vi "Build.vi"(8 "error in (no error)":errorcluster, 11 "CD Build Tools in":refnum<class "Project Sync Tools.lvclass">) -> (0 "error out":errorcluster, 3 "CD Build Tools out":refnum<class "Project Sync Tools.lvclass">)   [LabVIEW 2019]
uses:
  Project Sync Tools.lvclass
  <vilib>/AppBuilder/AB_API_Simple/NI_App_Builder_API.lvlib
  <vilib>/AppBuilder/AB_API_Simple/Build (path).vi
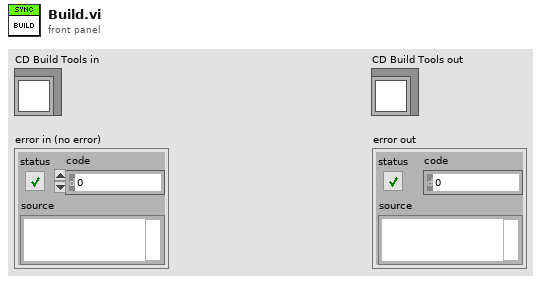
[diagram p1: front panel]
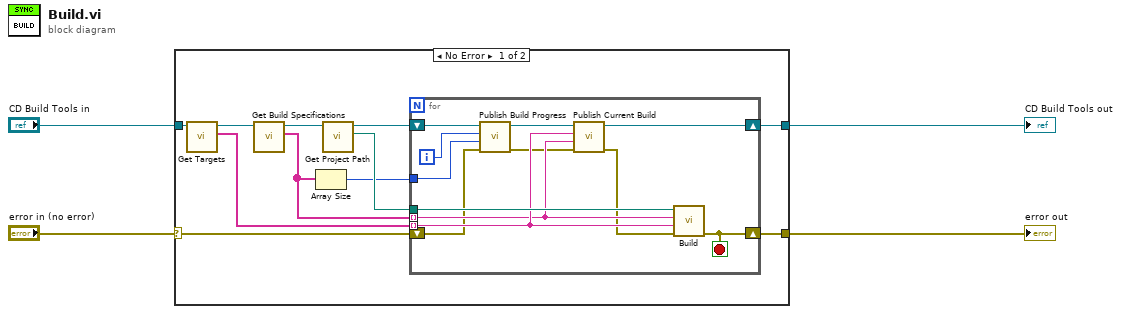
[diagram p0: block diagram]
diagram:
  n1 = case shown="No Error" "error in (no error)" {
    selector: "error in (no error)" -> [w9 w28]
    tunnel: [w5 w29] -> w1
    tunnel: [w13 w28] -> w2
    tunnel: "CD Build Tools in" -> [w12 w29]
    frame No Error {
      n2 = call "Get Targets.vi"("CD Build Tools in"=w12) -> ("Targets"=w10:string[], "CD Build Tools out"=w11:refnum<class "Project Sync Tools.lvclass">)  [unwired: 9 in]
      n3 = call "Get Build Specifications.vi"("CD Build Tools in"=w11) -> ("Build Specifications"=w8:string[], "CD Build Tools out"=w14:refnum<class "Project Sync Tools.lvclass">)  [unwired: 9 in]
      n4 = Array Size(array=w8) -> (size(s)=w7:i32)
      n5 = call "Get Project Path.vi"("CD Build Tools in"=w14) -> ("Project Path"=w15:path, "CD Build Tools out"=w6:refnum<class "Project Sync Tools.lvclass">)  [unwired: 9 in]
      n6 = for {
        tunnel: w15 -> [w27]
        shift-right: [w26] -> w13
        shift-left: w9 -> [w20]
        tunnel: w8 -> [w24] mode=indexing
        tunnel: w10 -> [w25] mode=indexing
        tunnel: w7 -> [w21]
        shift-right: [w17] -> w5
        shift-left: w6 -> [w23]
        i -> [w22]
        stop <- w26 stop-if-true
        n7 = call "Publish Build Progress.vi"("error in (no error)"=w20, "Total Number of Builds"=w21, "Current Iteration"=w22, "CD Build Tools in"=w23) -> ("error out"=w18:errorcluster, "CD Build Tools out"=w19:refnum<class "Project Sync Tools.lvclass">)  [unwired: 6 in]
        n8 = call "Publish Current Build.vi"("error in (no error)"=w18, "Build Specification Name"=w24, "Target"=w25, "CD Build Tools in"=w19) -> ("error out"=w16:errorcluster, "CD Build Tools out"=w17:refnum<class "Project Sync Tools.lvclass">)  [unwired: 6 in]
        n9 = call-poly <vilib>:"Build.vi"("error in (no error)"=w16, "Name of target (My Computer)"=w25, "Name of build specification (if empty: build all)"=w24, "Path to project"=w27) -> ("error out"=w26:errorcluster)  [unwired: 6 in, 1 out]
      }
    }
    frame Error {
    }
  }
  "error out" <- w2
  "CD Build Tools out" <- w1
